vi "Read Settings.vi"(8 "error in (no error)":errorcluster, 11 "Model in":refnum<class "Model.lvclass">) -> (0 "error out":errorcluster, 3 "Model out":refnum<class "Model.lvclass">)   [LabVIEW 2015, in "Model.lvclass"]
uses:
  Model.lvclass
  Boot Loader/Boot Loader.lvclass
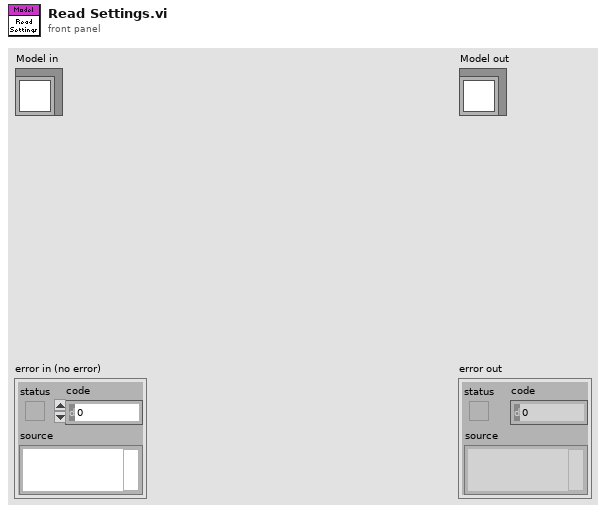
[diagram p1: front panel]
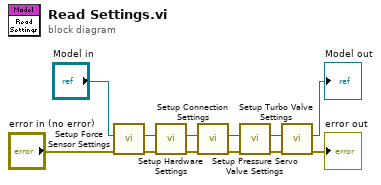
[diagram p0: block diagram]
diagram:
  n1 = call "Setup Force Sensor Settings.vi"("error in (no error)"="error in (no error)", "Model in"="Model in") -> ("error out"=w9:errorcluster, "Model out"=w10:refnum<class "Model.lvclass">)  [unwired: 7 in, 1 out]
  n2 = call "Setup Hardware Settings.vi"("error in (no error)"=w9, "Model in"=w10) -> ("error out"=w8:errorcluster, "Model out"=w7:refnum<class "Model.lvclass">)  [unwired: 7 in, 1 out]
  n3 = call "Setup Connection Settings.vi"("error in (no error)"=w8, "Model in"=w7) -> ("error out"=w5:errorcluster, "Model out"=w6:refnum<class "Model.lvclass">)  [unwired: 7 in, 1 out]
  n4 = call "Setup Pressure Servo Valve Settings.vi"("error in (no error)"=w5, "Model in"=w6) -> ("error out"=w4:errorcluster, "Model out"=w3:refnum<class "Model.lvclass">)  [unwired: 7 in, 1 out]
  n5 = call "Setup Turbo Valve Settings.vi"("error in (no error)"=w4, "Model in"=w3) -> ("error out"=→"error out":errorcluster, "Model out"=→"Model out":refnum<class "Model.lvclass">)  [unwired: 7 in, 1 out]
